vi "读取B版外设配置.vi"(8 "error in (no error)":errorcluster, 11 "MB session in":refnum<class "MB_Master.lvclass">) -> (0 "error out":errorcluster, 2 "外设配置":T1 {"阀型号" items=["垦拓10通阀"]; "总氮x公式0" items=["0", "1"]; "光谱仪类型" items=["1型", "2型", "3型", "2型氙灯联控"]; "泵阀量" items=["9通"=9, "10通"=10, "12通"=12]; "泵类型" items=["润泽注射泵", "垦拓注射泵"]}, 3 "MB session out":refnum<class "MB_Master.lvclass">)   [LabVIEW 2016, in "斯坦道总氮.lvlib"]
uses:
  <vilib>/Plasmionique/MB Master/MB_Master/MB_Master.lvclass
  <vilib>/Plasmionique/MB Master/MB_Master_Serial/MB_Master_Serial.lvclass
  C:/Program Files (x86)/National Instruments/LabVIEW 2016/vi.lib/Plasmionique/MB Master/MB_Master/MB_Master.lvclass
  <vilib>/Plasmionique/MB Master/MB Master.lvlib
panel:
  in  "VISA Resource":refnum<visa-resource-name>
  in  "引用选择":enum16{"MB引用", "自建引用"}(ring)
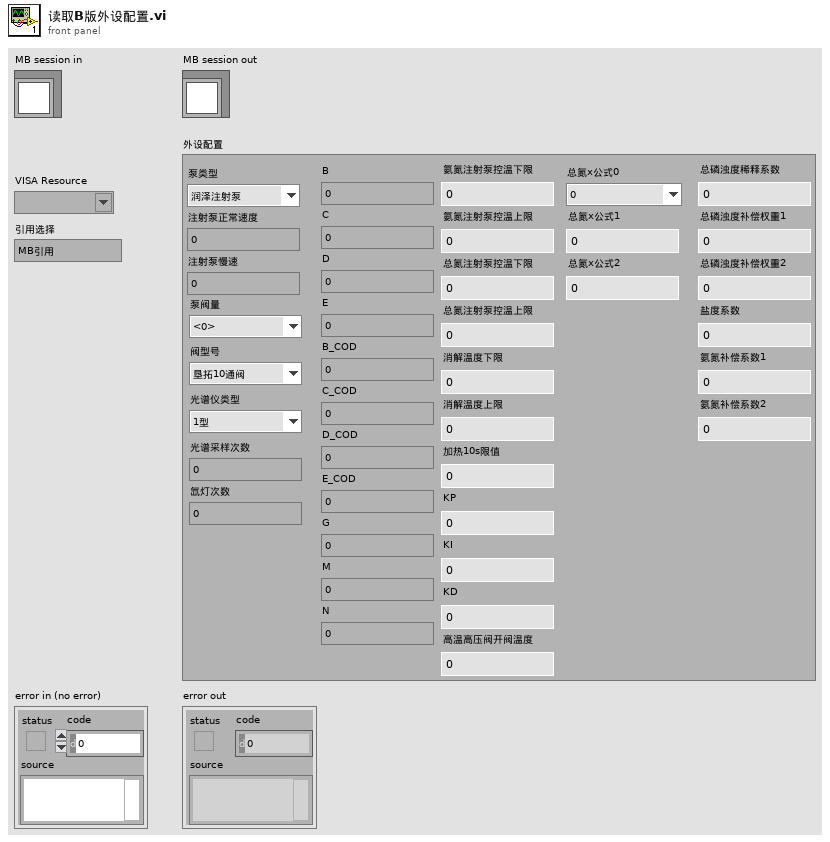
[diagram p1: front panel]
types:
  T1 = typedef "斯坦道总氮.lvlib/V3 B版外设参数.ctl" = cluster{"泵类型":u8, "注射泵正常速度":u32, "注射泵慢速":u32, "泵阀量":u8, "阀型号":u8, "光谱仪类型":u8, "光谱采样次数":u8, "氙灯次数":u8, "B":u16, "C":u16, "D":u16, "E":u16, "B_COD":u16, "C_COD":u16, "D_COD":u16, "E_COD":u16, "G":u16, "M":u16, "N":u16, "氨氮注射泵控温下限":sgl, "氨氮注射泵控温上限":sgl, "总氮注射泵控温下限":sgl, "总氮注射泵控温上限":sgl, "消解温度下限":sgl, "消解温度上限":sgl, "加热10s限值":sgl, "KP":sgl, "KI":sgl, "KD":sgl, "高温高压阀开阀温度":sgl, "总氮x公式0":u8, "总氮x公式1":sgl, "总氮x公式2":sgl, "总磷浊度稀释系数":sgl, "总磷浊度补偿权重1":sgl, "总磷浊度补偿权重2":sgl, "盐度系数":sgl, "氨氮补偿系数1":sgl, "氨氮补偿系数2":sgl}
  T2 = cluster{"baud rate (bps)":u32, "stop bits":u16, "parity":u16, "flow control":u16, "timeout":u32, "retries":i32}
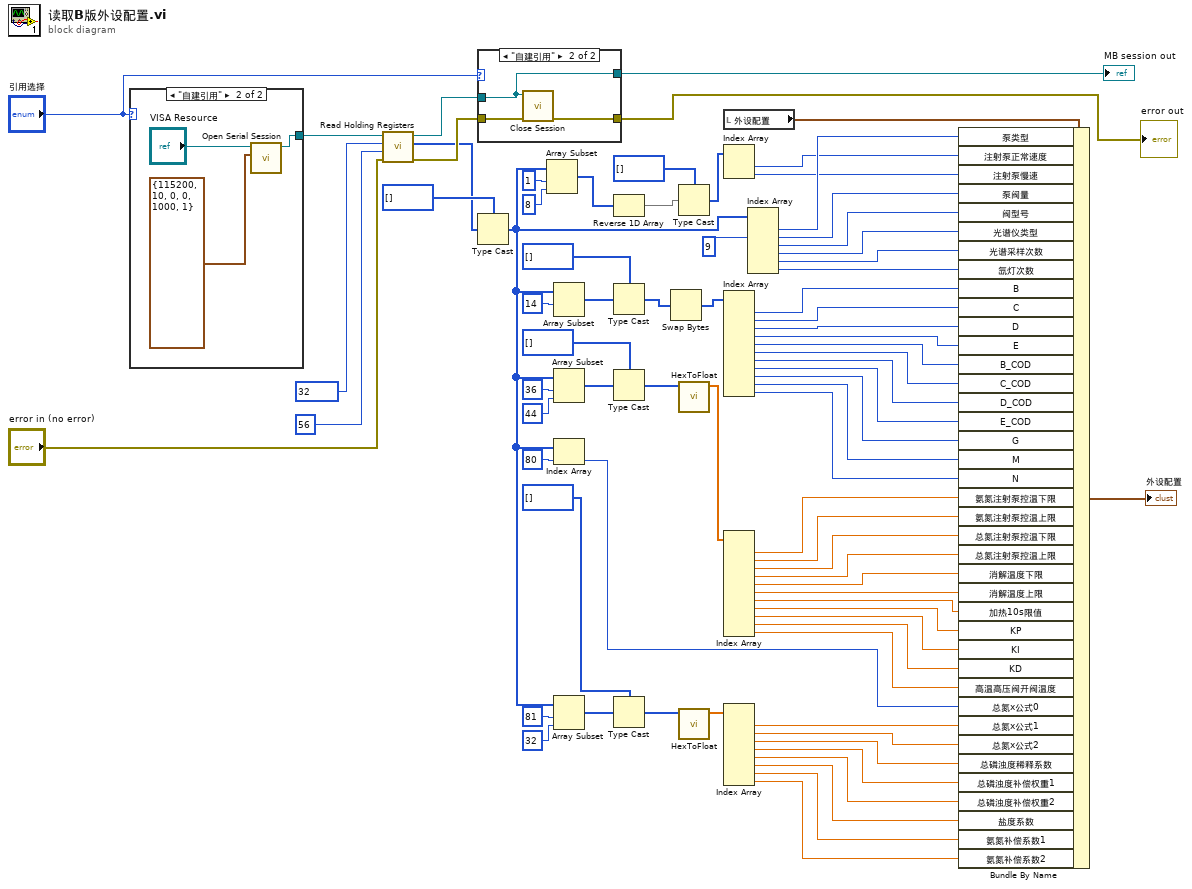
[diagram p0: block diagram]
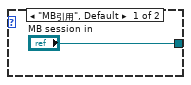
[diagram p3: hidden frame]
diagram:
  n1 = case shown="\"自建引用\"" "引用选择" {
    tunnel: ["MB session in" w82] -> w68
    frame "MB引用", Default {
    }
    frame "自建引用" {
      n2 = call <vilib>:"Open Serial Session.vi"("Serial Config"=T2 {"baud rate (bps)"=115200, "stop bits"=10, "parity"=0, "flow control"=0, "timeout"=1000, "retries"=1}, "VISA Resource"="VISA Resource") -> ("MB_Serial session"=w82:refnum<class "MB_Master_Serial.lvclass">)  [unwired: 8 in, 1 out]
    }
  }
  n3 = call <vilib>:"Read Holding Registers.vi"("error in (no error)"="error in (no error)", "quantity"=u16 56, "starting address"=u16 32, "MB session in"=w68) -> ("error out"=w65:errorcluster, "Registers"=w44:u16[], "MB session out"=w67:refnum<class "MB_Master.lvclass">)  [unwired: 5 in]
  n4 = case shown="\"自建引用\"" "引用选择" {
    tunnel: w67 -> [w83 w85]
    tunnel: w65 -> [w84 w87]
    tunnel: [w84 w86] -> w64
    tunnel: [w83 w85] -> w63
    frame "MB引用", Default {
    }
    frame "自建引用" {
      n5 = call-dynamic "Close Session.vi"("error in (no error)"=w87, "MB session in"=w85) -> ("error out"=w86:errorcluster)  [unwired: 9 in]
    }
  }
  "MB session out" <- w63
  "error out" <- w64
  n6 = Type Cast(type=u8[] [], x=w44) -> (*(type *) &x=w43:u8[])
  n7 = Array Subset(array=w43, index=1 ("索引"), length=8 ("长度")) -> (w72:u8[])
  n8 = Array Subset(array=w43, index=14 ("索引")) -> (w54:u8[])  [unwired: 1 in]
  n9 = Array Subset(array=w43, index=36 ("索引"), length=44 ("长度")) -> (w59:u8[])
  n10 = Index Array(array=w43, index=80 ("索引")) -> (element=w10:u8)
  n11 = Array Subset(array=w43, index=81 ("索引"), length=32 ("长度")) -> (w49:u8[])
  n12 = Reverse 1D Array(array=w72) -> (reversed array=w71:u8[])
  n13 = Type Cast(type=u16[] [], x=w54) -> (*(type *) &x=w53:u16[])
  n14 = Type Cast(type=u16[] [], x=w59) -> (*(type *) &x=w57:u16[])
  n15 = Type Cast(type=u16[] [], x=w49) -> (*(type *) &x=w48:u16[])
  n16 = Swap Bytes(anything=w53) -> (byte swapped=w52:u16[])
  n17 = Type Cast(type=u32[] [], x=w71) -> (*(type *) &x=w69:u32[])
  n18 = call "HexToFloat.vi"("数组"=w57) -> ("FLOAT"=w60:sgl[])  [unwired: 10 in]
  n19 = call "HexToFloat.vi"("数组"=w48) -> ("FLOAT"=w50:sgl[])  [unwired: 10 in]
  n20 = local read "外设配置"() -> (w42:T1)
  n21 = Index Array(array=w69) -> (element #1=w39:u32, element #2=w38:u32)  [unwired: 2 in]
  n22 = Index Array(array=w52) -> (element #1=w32:u16, element #2=w31:u16, element #3=w30:u16, element #4=w29:u16, element #5=w28:u16, element #6=w27:u16, element #7=w26:u16, element #8=w25:u16, element #9=w24:u16, element #10=w23:u16, element #11=w22:u16)  [unwired: 11 in]
  n23 = Index Array(array=w60) -> (element #1=w21:sgl, element #2=w20:sgl, element #3=w19:sgl, element #4=w18:sgl, element #5=w17:sgl, element #6=w16:sgl, element #7=w15:sgl, element #8=w14:sgl, element #9=w13:sgl, element #10=w12:sgl, element #11=w11:sgl)  [unwired: 11 in]
  n24 = Index Array(array=w50) -> (element #1=w9:sgl, element #2=w8:sgl, element #3=w7:sgl, element #4=w6:sgl, element #5=w5:sgl, element #6=w4:sgl, element #7=w3:sgl, element #8=w2:sgl)  [unwired: 8 in]
  n25 = Index Array(array=w43, index #2=9 ("索引")) -> (element #1=w40:u8, element #2=w37:u8, element #3=w36:u8, element #4=w35:u8, element #5=w34:u8, element #6=w33:u8)  [unwired: 5 in]
  n26 = Bundle By Name(cluster=w42, "泵类型"=w40, "注射泵正常速度"=w39, "注射泵慢速"=w38, "泵阀量"=w37, "阀型号"=w36, "光谱仪类型"=w35, "光谱采样次数"=w34, "氙灯次数"=w33, "B"=w32, "C"=w31, "D"=w30, "E"=w29, "B_COD"=w28, "C_COD"=w27, "D_COD"=w26, "E_COD"=w25, "G"=w24, "M"=w23, "N"=w22, "氨氮注射泵控温下限"=w21, "氨氮注射泵控温上限"=w20, "总氮注射泵控温下限"=w19, "总氮注射泵控温上限"=w18, "消解温度下限"=w17, "消解温度上限"=w16, "加热10s限值"=w15, "KP"=w14, "KI"=w13, "KD"=w12, "高温高压阀开阀温度"=w11, "总氮x公式0"=w10, "总氮x公式1"=w9, "总氮x公式2"=w8, "总磷浊度稀释系数"=w7, "总磷浊度补偿权重1"=w6, "总磷浊度补偿权重2"=w5, "盐度系数"=w4, "氨氮补偿系数1"=w3, "氨氮补偿系数2"=w2) -> (→"外设配置":T1)
